vi "Compare Waveform Stream Specifications.vi"(8 "error in (no error)":errorcluster, 10 "WaveformStreamSpecification to compare":T1, 11 "WaveformStreamSpecification":T1) -> (0 "error out":errorcluster, 3 "equivalent?":bool)   [LabVIEW 2020, in "NI_VS Waveform Streaming Interface.lvlib"]
doc: "Compares two waveform stream specifications to see if they define the same streaming operation. This VI compares the waveform paths, streaming rates, and conditions under which to stream data for the waveforms."
uses:
  <vilib>/NI VeriStand/Execution/WaveformStreaming/NI_VS Waveform Streaming Interface.lvlib
  <vilib>/NI VeriStand/Execution/WaveformStreaming/WaveformStreamSpecification.ctl
  NationalInstruments.VeriStand.ClientAPI
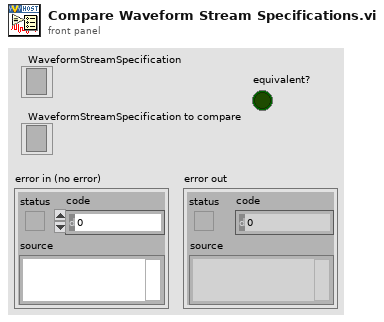
[diagram p1: front panel]
types:
  T1 = typedef "NI_VS Waveform Streaming Interface.lvlib/WaveformStreamSpecification.ctl" = refnum<k24>
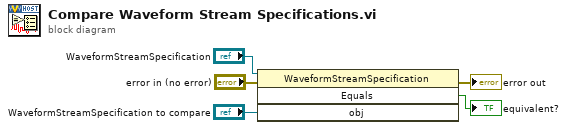
[diagram p0: block diagram]
diagram:
  n1 = invoke class="WaveformStreamSpecification" method="Equals"(reference="WaveformStreamSpecification", error in="error in (no error)", "obj"="WaveformStreamSpecification to compare") -> (error out=→"error out":errorcluster, "Equals"=→"equivalent?":bool)  [unwired: 1 in, 2 out]
